vi "present_current.vi"() -> ()   [LabVIEW 2013]
panel:
  out "Present I (mA)":dbl=0.2362
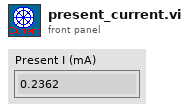
[diagram p1: front panel]
diagram:
